vi "Run Bfr Rx - Sized Write Buffer.vi"(4 "Data Buffer":u64, 6 "Data":u8[](array[numeric]), 7 "Size Offset in":u64, 8 "error in (no error)":errorcluster, 10 "Null Offset in":u64, 11 "Data Offset in":u64) -> (0 "error out":errorcluster)   [LabVIEW 2019, in "UDP-Custom-Device Engine.lvlib"]
uses:
  UDP-Custom-Device Engine.lvlib
  <vilib>/NI VeriStand/VeriStand Data/Pointer Operations/Pointer.Write (1D U8).vi
  <vilib>/NI VeriStand/VeriStand Data/Pointer Operations/Pointer.Write (I32).vi
  <vilib>/NI VeriStand/VeriStand Data/VeriStand Data.lvlib
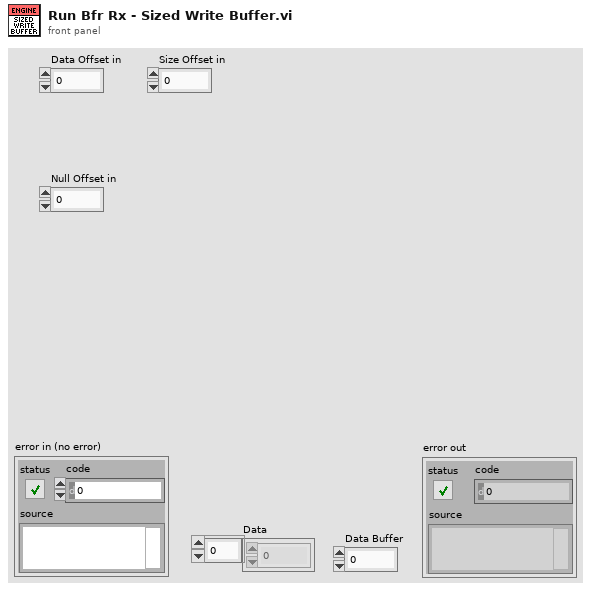
[diagram p1: front panel]
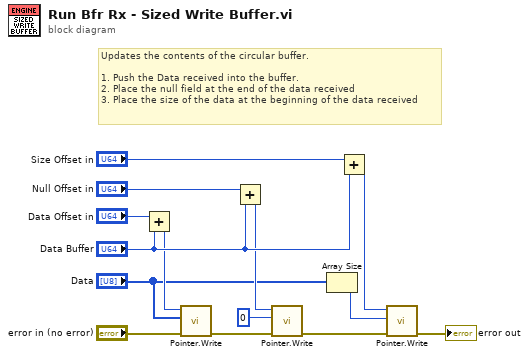
[diagram p0: block diagram]
diagram:
  # "Updates the contents of the circular buffer.\n\n1. Push the Data received into the buffer.\n2. Place the null field at the end of the data received\n3. Place the size of the data at the beginning of the data received"
  n1 = Add(x="Data Offset in", y="Data Buffer") -> (x+y=w6:u64)
  n2 = call-poly <vilib>:"Pointer.Write.vi"("error in (no error)"="error in (no error)", "values"="Data", "pointer in"=w6) -> ("error out"=w3:errorcluster)  [unwired: 6 in, 2 out]
  n3 = Add(x="Null Offset in", y="Data Buffer") -> (x+y=w8:u64)
  n4 = call-poly <vilib>:"Pointer.Write.vi"("error in (no error)"=w3, "value"=0, "pointer in"=w8) -> ("error out"=w2:errorcluster)  [unwired: 6 in, 2 out]
  n5 = Array Size(array="Data") -> (size(s)=w9:i32)
  n6 = Add(x="Size Offset in", y="Data Buffer") -> (x+y=w10:u64)
  n7 = call-poly <vilib>:"Pointer.Write.vi"("error in (no error)"=w2, "value"=w9, "pointer in"=w10) -> ("error out"=→"error out":errorcluster)  [unwired: 6 in, 2 out]
